vi "整合-测量信息至列表框.vi"(2 "报警方式":T1(array[cluster]), 4 "限值":T3(array[cluster]), 5 "累积剂量":T2(array[cluster]), 6 "测量值":cluster{"X":timestamp, "Y":dbl}[](array[cluster]), 7 "MCListbox引用句柄":refnum<vi>, 8 "备注信息":string[](array[string]), 9 "报警状态":enum16{"正常", "一级报警", "二级报警", "累积报警"}[](array[ring]), 10 "探头地址":i32[](array[numeric]), 11 "探头启用状态？":bool[](array[boolean])) -> (3 "报警状态状态":enum16{"正常", "一级报警", "二级报警", "累积报警"}(ring))   [LabVIEW 2017]
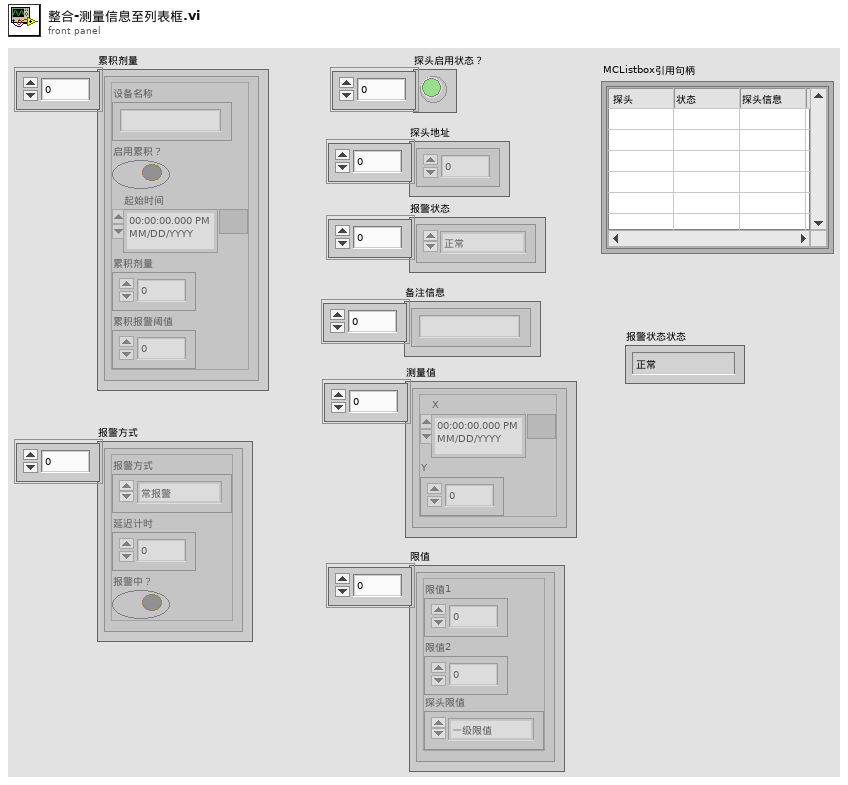
[diagram p1: front panel]
types:
  T1 = cluster{"报警方式":enum16{"常报警", "自动静音", "手动静音"}, "延迟计时":u16, "报警中？":bool}[]
  T2 = cluster{"设备名称":string, "启用累积？":bool, "起始时间":timestamp, "累积剂量":dbl, "累积报警阈值":dbl}[]
  T3 = cluster{"限值1":dbl, "限值2":dbl, "探头限值":enum16{"一级限值", "二级限值"}}[]
  T4 = cluster{"设备名称":string, "启用累积？":bool, "起始时间":timestamp, "累积剂量":dbl, "累积报警阈值":dbl}
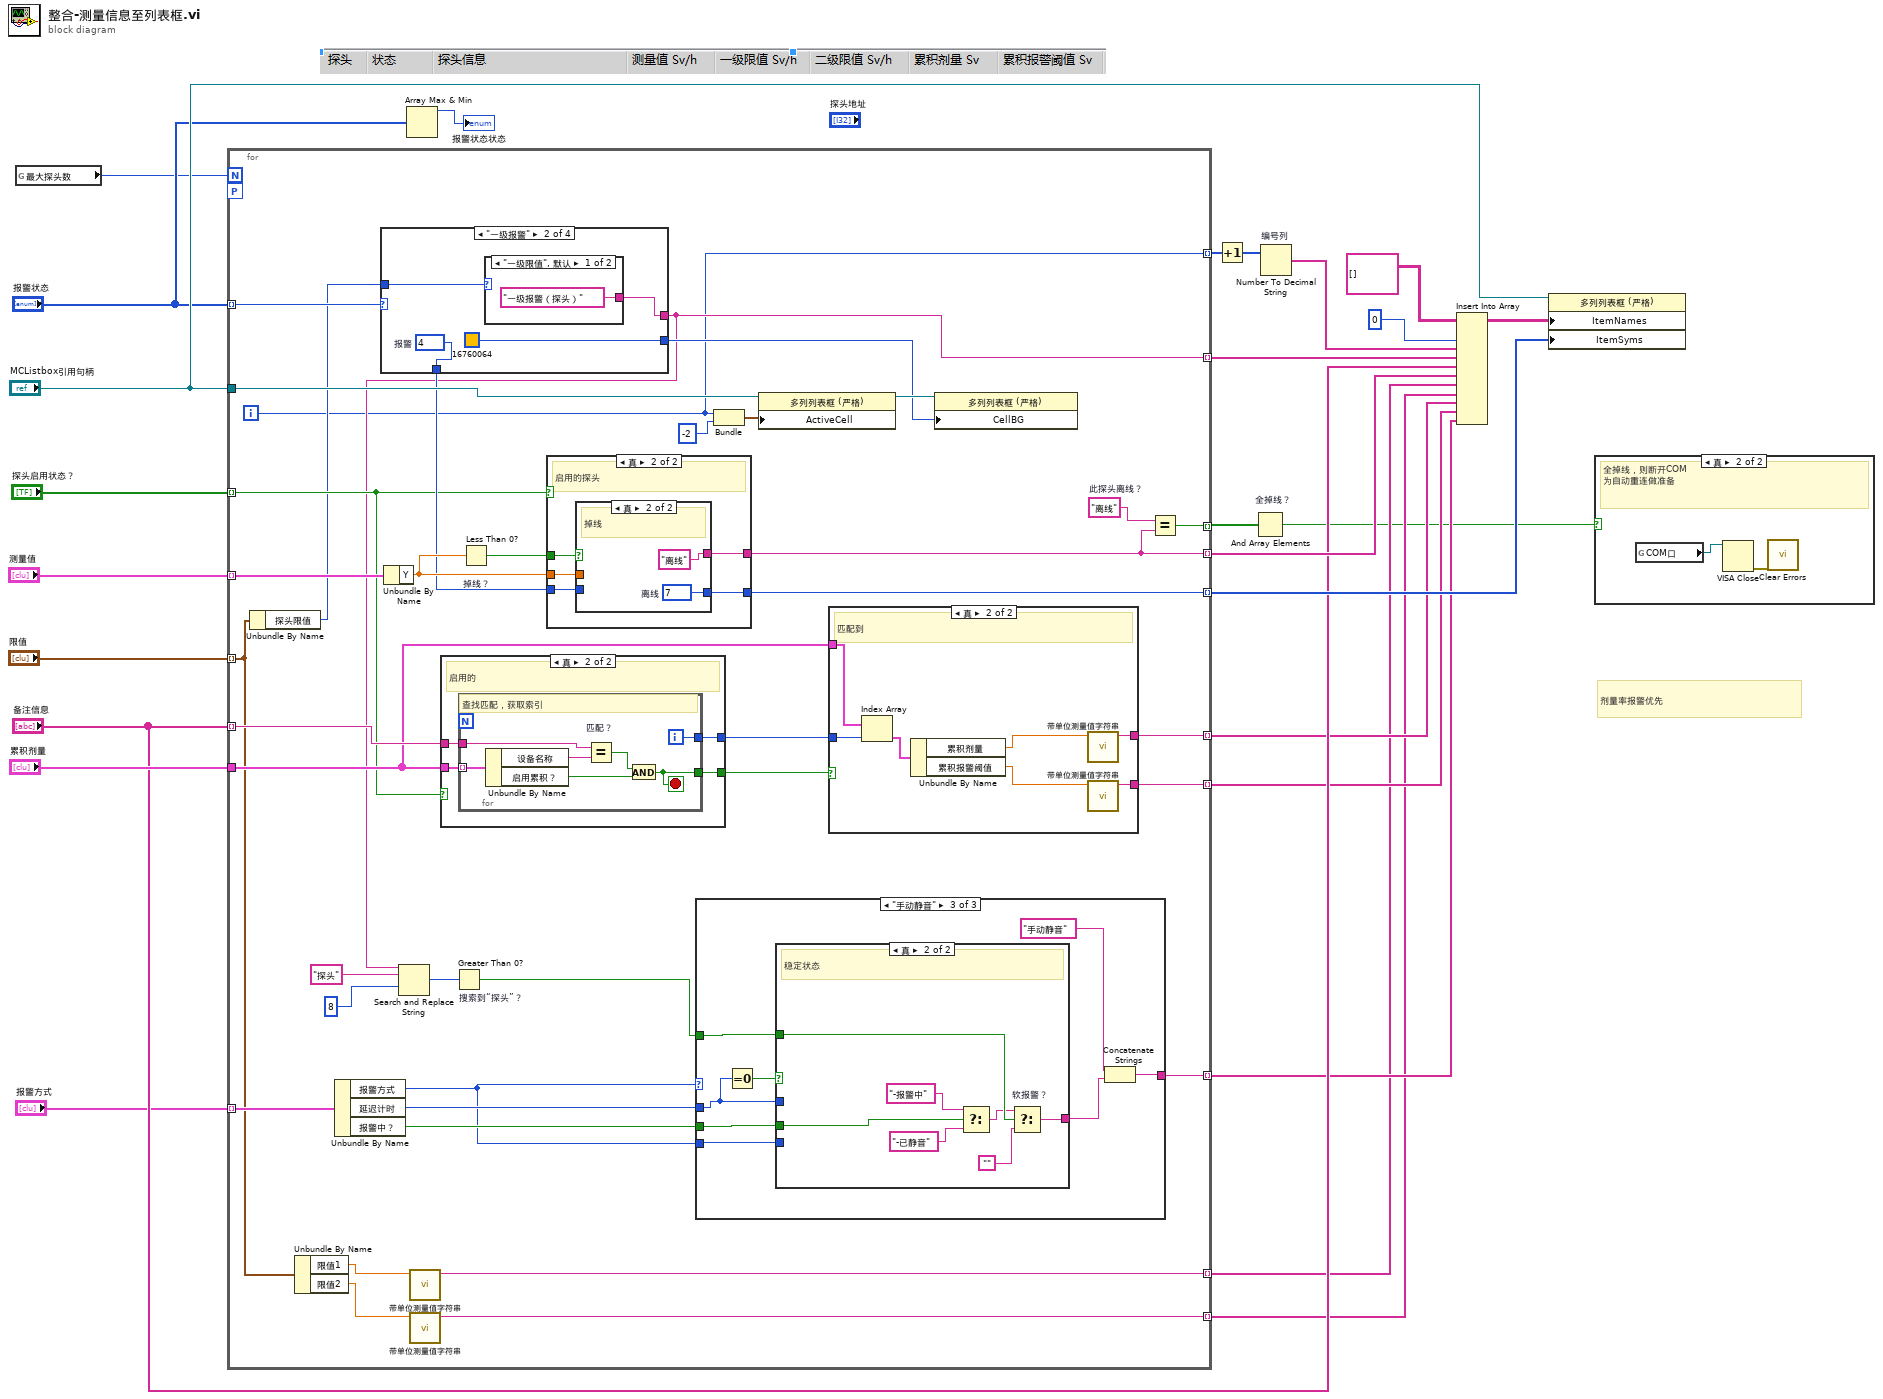
[diagram p0: block diagram]
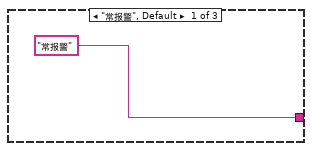
[diagram p3: hidden frame]
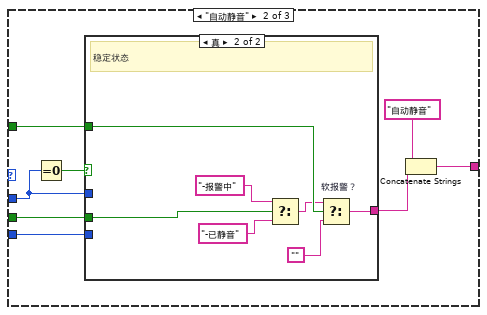
[diagram p4: hidden frame]
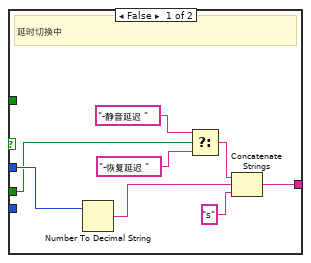
[diagram p5: hidden frame]
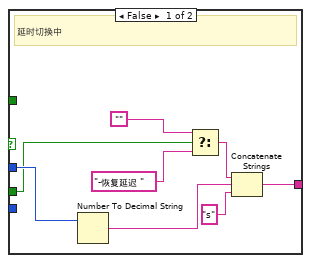
[diagram p6: hidden frame]
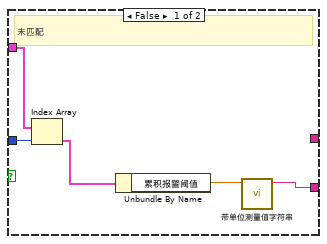
[diagram p8: hidden frame]
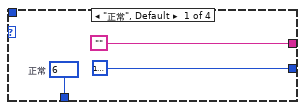
[diagram p9: hidden frame]
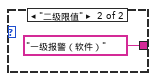
[diagram p10: hidden frame]
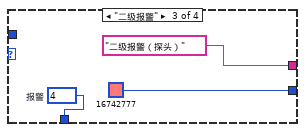
[diagram p11: hidden frame]
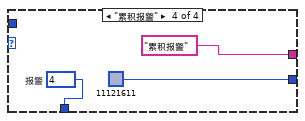
[diagram p12: hidden frame]
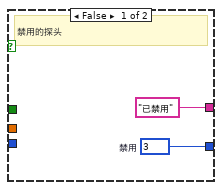
[diagram p13: hidden frame]
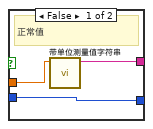
[diagram p14: hidden frame]
diagram:
  # "剂量率报警优先"
  n1 = global read "全局变量-35点监测.vi" "最大探头数"() -> (w1:i32)
  n2 = for {
    N: w1 -> [_]
    tunnel: "报警状态" -> [w45] mode=indexing
    tunnel: "测量值" -> [w59] mode=indexing
    tunnel: [w30] -> w18 mode=indexing
    tunnel: "MCListbox引用句柄" -> [w61]
    tunnel: "探头启用状态？" -> [w48] mode=indexing
    workers-P: _ -> [_]
    tunnel: [w35] -> w19 mode=indexing
    tunnel: [w49] -> w14 mode=indexing
    tunnel: "累积剂量" -> [w54]
    tunnel: "备注信息" -> [w55] mode=indexing
    tunnel: [w52] -> w11 mode=indexing
    tunnel: [w51] -> w10 mode=indexing
    tunnel: "报警方式" -> [w47] mode=indexing
    tunnel: [w43] -> w8 mode=indexing
    tunnel: "限值" -> [w40] mode=indexing
    tunnel: [w37] -> w6 mode=indexing
    tunnel: [w36] -> w5 mode=indexing
    tunnel: [w27] -> w4 mode=indexing
    tunnel: [w28] -> w3 mode=indexing
    i -> [w27]
    w29 = "离线"  # 此探头离线？
    n3 = Unbundle By Name(w40) -> ("探头限值"=w41:enum16{"一级限值", "二级限值"})
    n4 = Unbundle By Name(w40) -> ("限值1"=w39:dbl, "限值2"=w38:dbl)
    n5 = Unbundle By Name(w47) -> ("报警方式"=w42:enum16{"常报警", "自动静音", "手动静音"}, "延迟计时"=w44:u16, "报警中？"=w46:bool)
    n6 = case shown="\"一级报警\"" w45 {
      tunnel: [u32 16777226 u32 16760064 u32 16742777 u32 11121611] -> w57
      tunnel: ["" w138 "二级报警（探头）" ("数值输入控件") "累积报警" ("数值输入控件")] -> w35
      tunnel: [w135 w140 w145 w148] -> w56
      tunnel: w41 -> [_ w139 _ _]
      frame "正常", Default {
        w135 = 6  # 正常
      }
      frame "一级报警" {
        w140 = 4  # 报警
        n7 = case shown="\"一级限值\", 默认" w139 {
          tunnel: ["一级报警（探头）" ("数值输入控件") "一级报警（软件）" ("数值输入控件")] -> w138
          frame "一级限值", Default {
          }
          frame "二级限值" {
          }
        }
      }
      frame "二级报警" {
        w145 = 4  # 报警
      }
      frame "累积报警" {
        w148 = 4  # 报警
      }
    }
    n8 = Unbundle By Name(w59) -> ("Y"=w58:dbl)
    n9 = Search and Replace String(input string=w35, search string="探头" ("正则表达式"), offset=8 ("偏移量(0)")) -> (number of replacements=w32:i32)  [unwired: 5 in, 3 out]
    n10 = call "带单位测量值字符串.vi"("测量值"=w39) -> ("结果"=w37:string)  [unwired: 10 in]
    n11 = call "带单位测量值字符串.vi"("测量值"=w38) -> ("结果"=w36:string)  [unwired: 10 in]
    n12 = case shown="真" w48 {
      tunnel: w55 -> [_ w115]
      tunnel: w54 -> [_ w114]
      tunnel: [_ w113] -> w53
      tunnel: [_ w112] -> w50
      frame False {
        # "未启用"
      }
      frame True {
        # "启用的"
        n13 = for {
          tunnel: w114 -> [w122] mode=indexing
          tunnel: w115 -> [w120]
          tunnel: [w117] -> w113
          tunnel: [w116] -> w112
          i -> [w117]
          stop <- w116 stop-if-true
          # "查找匹配，获取索引"
          n14 = Unbundle By Name(w122) -> ("设备名称"=w121:string, "启用累积？"=w118:bool)
          n15 = Equal? "匹配？"(x=w120, y=w121) -> (x = y?=w119:bool)
          n16 = And(x=w119, y=w118) -> (x .and. y?=w116:bool)
        }
      }
    }
    n17 = Greater Than 0? "搜索到“探头”？"(x=w32) -> (x > 0?=w31:bool)
    n18 = Less Than 0? "掉线？"(x=w58) -> (x < 0?=w62:bool)
    n19 = case shown="真" w48 {
      tunnel: w62 -> [_ w156]
      tunnel: w58 -> [_ w155]
      tunnel: ["已禁用" ("数值输入控件") w154] -> w30
      tunnel: [w150 w153] -> w49
      tunnel: w56 -> [_ w152]
      frame False {
        w150 = 3  # 禁用
        # "禁用的探头"
      }
      frame True {
        # "启用的探头"
        n20 = case shown="真" w156 {
          tunnel: [w158 "离线" ("数值输入控件")] -> w154
          tunnel: w155 -> [w159 _]
          tunnel: [w157 w160] -> w153
          tunnel: w152 -> [w157 _]
          frame False {
            # "正常值"
            n21 = call "带单位测量值字符串.vi"("测量值"=w159) -> ("结果"=w158:string)  [unwired: 10 in]
          }
          frame True {
            w160 = 7  # 离线
            # "掉线"
          }
        }
      }
    }
    n22 = case shown="\"手动静音\"" w42 {
      tunnel: w46 -> [_ w72 w91]
      tunnel: w44 -> [_ w71 w92]
      tunnel: w42 -> [_ w69 w90]
      tunnel: ["常报警" w68 w89] -> w43
      tunnel: w31 -> [_ w66 w93]
      frame "常报警", Default {
      }
      frame "自动静音" {
        n23 = Equal To 0?(x=w71) -> (x = 0?=w73:bool)
        n24 = case shown="真" w73 {
          tunnel: w72 -> [w74 w88]
          tunnel: w71 -> [w79 _]
          tunnel: [w75 w82] -> w70
          tunnel: w69 -> [_ _]
          tunnel: w66 -> [_ w85]
          frame False {
            # "延时切换中"
            n25 = Number To Decimal String(number=w79) -> (decimal integer string=w77:string)  [unwired: 1 in]
            n26 = Select(t="-静音延迟 ", s=w74, f="-恢复延迟 ") -> (s? t:f=w78:string)
            n27 = Concatenate Strings(w78, w77, "s") -> (w75:string)
          }
          frame True {
            # "稳定状态"
            n28 = Select(t="-报警中", s=w88, f="-已静音") -> (s? t:f=w84:string)
            n29 = Select "软报警？"(t=w84, s=w85, f="") -> (s? t:f=w82:string)
          }
        }
        n30 = Concatenate Strings("自动静音", w70) -> (w68:string)
      }
      frame "手动静音" {
        n31 = Equal To 0?(x=w92) -> (x = 0?=w96:bool)
        n32 = case shown="真" w96 {
          tunnel: w91 -> [w97 w111]
          tunnel: w92 -> [w102 _]
          tunnel: [w98 w105] -> w95
          tunnel: w90 -> [_ _]
          tunnel: w93 -> [_ w108]
          frame False {
            # "延时切换中"
            n33 = Number To Decimal String(number=w102) -> (decimal integer string=w100:string)  [unwired: 1 in]
            n34 = Select(t="", s=w97, f="-恢复延迟 ") -> (s? t:f=w101:string)
            n35 = Concatenate Strings(w101, w100, "s") -> (w98:string)
          }
          frame True {
            # "稳定状态"
            n36 = Select(t="-报警中", s=w111, f="-已静音") -> (s? t:f=w107:string)
            n37 = Select "软报警？"(t=w107, s=w108, f="") -> (s? t:f=w105:string)
          }
        }
        n38 = Concatenate Strings("手动静音", w95) -> (w89:string)
      }
    }
    n39 = Bundle(w27, -2) -> (w63:cluster{i32, i32})  [unwired: 1 in]
    n40 = property class="多列列表框 (严格)"(reference=w61, "ActiveCell"=w63) -> (reference out=w60:refnum<vi>)  [unwired: 1 in, 1 out]
    n41 = case shown="真" w50 {
      tunnel: w54 -> [w124 w134]
      tunnel: w53 -> [w123 w133]
      tunnel: [_ w131] -> w52
      tunnel: [w125 w130] -> w51
      frame False {
        # "未匹配"
        n42 = Index Array(array=w124, index=w123) -> (element=w127:T4)
        n43 = Unbundle By Name(w127) -> ("累积报警阈值"=w126:dbl)
        n44 = call "带单位测量值字符串.vi"("测量值"=w126) -> ("结果"=w125:string)  [unwired: 10 in]
      }
      frame True {
        # "匹配到"
        n45 = Index Array(array=w134, index=w133) -> (element=w132:T4)
        n46 = Unbundle By Name(w132) -> ("累积剂量"=w129:dbl, "累积报警阈值"=w128:dbl)
        n47 = call "带单位测量值字符串.vi"("测量值"=w129) -> ("结果"=w131:string)  [unwired: 10 in]
        n48 = call "带单位测量值字符串.vi"("测量值"=w128) -> ("结果"=w130:string)  [unwired: 10 in]
      }
    }
    n49 = property class="多列列表框 (严格)"(reference=w60, "CellBG"=w57) -> ()  [unwired: 1 in, 2 out]
    n50 = Equal?(x=w29, y=w30) -> (x = y?=w28:bool)
  }
  n51 = Array Max & Min(array="报警状态") -> (max value=→"报警状态状态":enum16{"正常", "一级报警", "二级报警", "累积报警"})  [unwired: 3 out]
  n52 = Increment(x=w4) -> (x+1=w15:i32[])
  n53 = And Array Elements "全掉线？"(Boolean array=w3) -> (logical AND=w2:bool)
  n54 = Number To Decimal String "编号列"(number=w15) -> (decimal integer string=w20:string[])  [unwired: 1 in]
  n55 = Insert Into Array(array=string[][] [] ("十进制整型字符串"), index (col)=0 ("禁用的索引 (列)"), new element #1=w20, new element #2=w19, new element #3="备注信息", new element #4=w18, new element #5=w6, new element #6=w5, new element #7=w11, new element #8=w10, new element #9=w8) -> (w24:string[][])  [unwired: 1 in]
  n56 = property class="多列列表框 (严格)"(reference="MCListbox引用句柄", "ItemNames"=w24, "ItemSyms"=w14) -> ()  [unwired: 1 in, 2 out]
  n57 = case shown="真" w2 {
    frame False {
    }
    frame True {
      # "全掉线，则断开COM\n为自动重连做准备"
      n58 = global read "全局变量-35点监测.vi" "COM口"() -> (w163:refnum<visa-resource-name>)
      n59 = VISA Close(VISA resource name=w163) -> (error out=w162:errorcluster)  [unwired: 1 in]
      n60 = call <vilib>:"Clear Errors.vi"("error in (no error)"=w162) -> ()  [unwired: 5 in, 2 out]
    }
  }
